vi "Test Create (From State String Constant).vi"(8 "error in (no error)":errorcluster) -> (0 "error out":errorcluster)   [LabVIEW 2013, in "TEST JKI State Machine API.lvlib"]
uses:
  TEST JKI State Machine API.lvlib
  <vilib>/addons/_JKI Toolkits/Caraya/classes/Assert/Assert.lvclass
  <vilib>/addons/_JKI Toolkits/Caraya/classes/Test/Test.lvclass
  source/JKI SM/JKI SM.lvclass
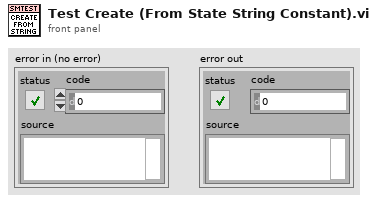
[diagram p1: front panel]
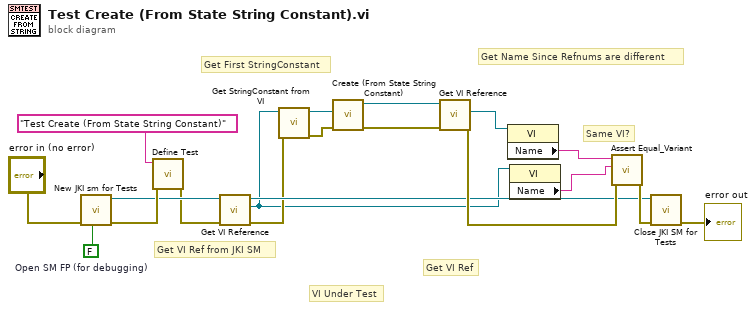
[diagram p0: block diagram]
diagram:
  w5 = FALSE  # Open SM FP (for debugging)
  # "Get Name Since Refnums are different"
  # "Get VI Ref"
  # "VI Under Test"
  # "Get First StringConstant"
  # "Same VI?"
  # "Get VI Ref from JKI SM"
  n1 = call "New JKI sm for Tests.vi"("Open SM FP (for debugging)"=w5, "error in (no error)"="error in (no error)") -> ("error out"=w19:errorcluster, "JKI SM out"=w14:refnum<class "JKI SM.lvclass">)  [unwired: 8 in]
  n2 = call <vilib>:"Define Test.vi"("error in (no error)"=w19, "Label (VI Title)"="Test Create (From State String Constant)") -> ("error out"=w13:errorcluster)  [unwired: 9 in]
  n3 = call "Get VI Reference.vi"("error in (no error)"=w13, "JKI SM in"=w14) -> ("error out"=w7:errorcluster, "VI"=w2:refnum<vi>, "JKI SM out"=w10:refnum<class "JKI SM.lvclass">)  [unwired: 7 in]
  n4 = call "Get StringConstant from VI.vi"("error in (no error)"=w7, "VI in"=w2) -> ("error out"=w6:errorcluster, "StringConstant out"=w8:refnum<vi>)  [unwired: 8 in]
  n5 = call "Create (From State String Constant).vi"("error in (no error)"=w6, "State String Constant"=w8) -> ("error out"=w12:errorcluster, "JKI SM out"=w9:refnum<class "JKI SM.lvclass">)  [unwired: 6 in, 2 out]
  n6 = call "Get VI Reference.vi"("error in (no error)"=w12, "JKI SM in"=w9) -> ("error out"=w11:errorcluster, "VI"=w4:refnum<vi>)  [unwired: 7 in, 1 out]
  n7 = property class="VI"(reference=w4) -> ("Name"=w3:string)  [unwired: 1 in, 2 out]
  n8 = property class="VI"(reference=w2) -> ("Name"=w1:string)  [unwired: 1 in, 2 out]
  n9 = call <vilib>:"Assert Equal_Variant.vi"("error in (no error)"=w11, "Y"=w1, "X"=w3) -> ("error out"=w16:errorcluster)  [unwired: 8 in]
  n10 = call "Close JKI SM for Tests.vi"("error in (no error)"=w16, "JKI SM in"=w10) -> ("error out"=→"error out":errorcluster)  [unwired: 9 in]
